vi "方程子VI3.vi"(8 "X":dbl, 9 "C":dbl, 10 "B":dbl, 11 "A":dbl) -> (2 "输出变量":dbl)   [LabVIEW 2018]
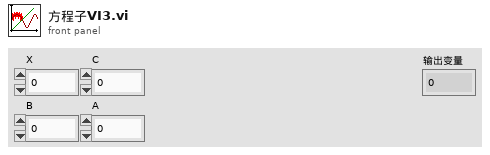
[diagram p1: front panel]
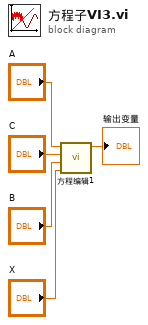
[diagram p0: block diagram]
diagram:
  n1 = call "方程编辑1.vi"("X"="X", "B"="B", "C"="C", "A"="A") -> ("输出变量"=→"输出变量":dbl)  [unwired: 7 in]
